vi "Anaylse.vi"(8 "error in (no error)":errorcluster, 10 "ImageData":T1, 11 "AbsorptionAnalyser in":refnum<class "AbsorptionAnalyser.lvclass">) -> (0 "error out":errorcluster, 3 "AbsorptionAnalyser out":refnum<class "AbsorptionAnalyser.lvclass">)   [LabVIEW 2009, in "Tools.lvlib" / "Imaging.lvlib" / "AbsorptionAnalyser.lvclass"]
uses:
  AbsorptionAnalyser.lvclass
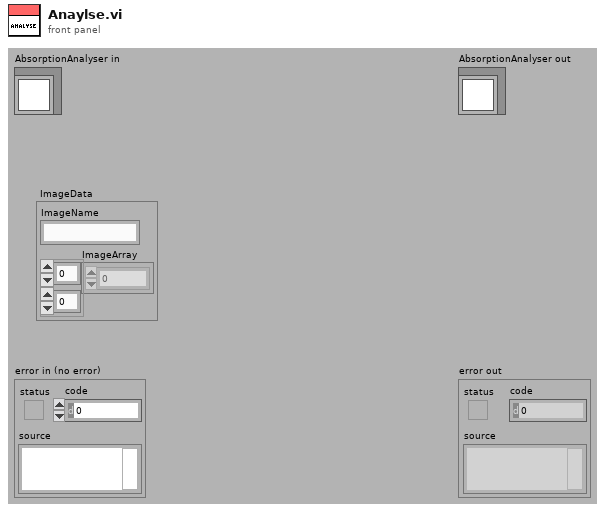
[diagram p1: front panel]
types:
  T1 = cluster{"ImageName":string, "ImageArray":sgl[][]}
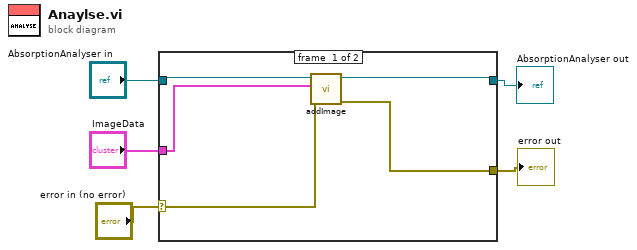
[diagram p0: block diagram]
diagram:
  n1 = case shown="No Error" "error in (no error)" {
    selector: "error in (no error)" -> [w8 w11]
    tunnel: [w7 w11] -> w4
    tunnel: [w9 w12] -> w3
    tunnel: "AbsorptionAnalyser in" -> [w10 w12]
    tunnel: "ImageData" -> [w6 _]
    frame #0 {
      n2 = call "addImage.vi"("error in (no error)"=w8, "ImageData"=w6, "AbsorptionAnalyser in"=w10) -> ("error out"=w7:errorcluster, "AbsorptionAnalyser out"=w9:refnum<class "AbsorptionAnalyser.lvclass">)  [unwired: 7 in]
    }
    frame #1 {
    }
  }
  "error out" <- w4
  "AbsorptionAnalyser out" <- w3
